vi "Divide into Input and Output.vi"(0 "front pane objects":refnum<vi>[](array[refnum])) -> (1 "objects 1":refnum<vi>[](array[refnum]), 2 "objects 2":refnum<vi>[](array[refnum]))   [LabVIEW 2016]
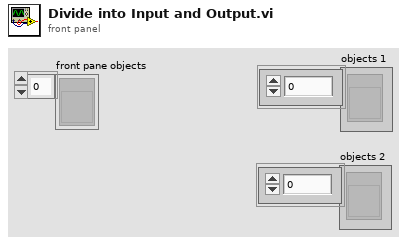
[diagram p1: front panel]
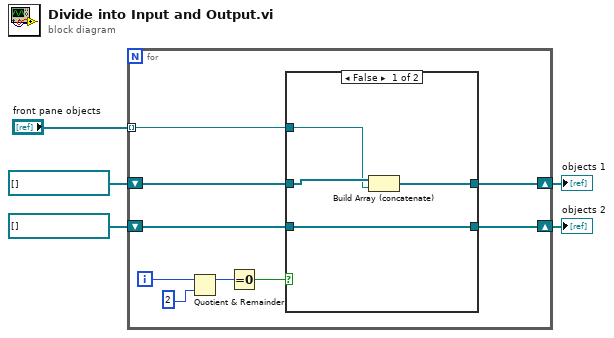
[diagram p0: block diagram]
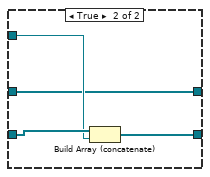
[diagram p2: hidden frame]
diagram:
  n1 = for {
    tunnel: "front pane objects" -> [w10] mode=indexing
    shift-right: [w8] -> w1
    shift-left: refnum<vi>[] [] ("All Objects[]") -> [w9]
    shift-right: [w7] -> w2
    shift-left: refnum<vi>[] [] ("All Objects[]") -> [w12]
    i -> [w14]
    n2 = Quotient & Remainder(x=w14, y=2) -> (x-y*floor(x/y)=w6:i32)  [unwired: 1 out]
    n3 = Equal To 0?(x=w6) -> (x = 0?=w11:bool)
    n4 = case shown="False" w11 {
      tunnel: w12 -> [w18 w19]
      tunnel: w10 -> [w17 w21]
      tunnel: w9 -> [w15 w22]
      tunnel: [w15 w20] -> w8
      tunnel: [w16 w19] -> w7
      frame False {
        n5 = Build Array (concatenate)(w18, w17) -> (w16:refnum<vi>[])
      }
      frame True {
        n6 = Build Array (concatenate)(w22, w21) -> (w20:refnum<vi>[])
      }
    }
  }
  "objects 1" <- w2
  "objects 2" <- w1
